vi "Emergency stop (SILAR).vi"(8 "error in":errorcluster, 10 "Аварийная остановка":bool, 11 "Arduino Resource In":T1={"VISA resource"="", "Board Type"=enum."Uno", "Connection Type"=enum."USB / Serial", "Bytes Per Packet (15)"=15}) -> (0 "error out":errorcluster, 3 "Arduino Resource Out":T1={"VISA resource"="", "Board Type"=enum."Uno", "Connection Type"=enum."USB / Serial", "Bytes Per Packet (15)"=15})   [LabVIEW 2012]
uses:
  <vilib>/LabVIEW Interface for Arduino/Type Defs/Arduino Resource.ctl
  <vilib>/LabVIEW Interface for Arduino/Type Defs/Board Type.ctl
  <vilib>/LabVIEW Interface for Arduino/LabVIEW Interface for Arduino.lvlib
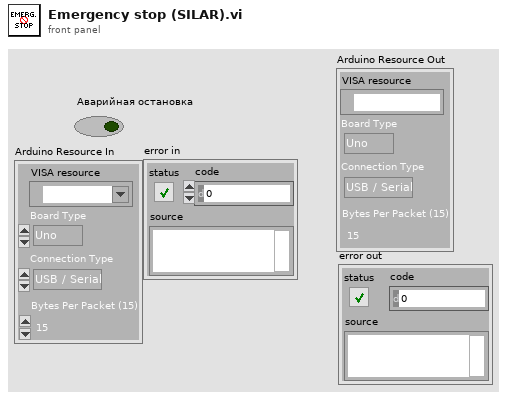
[diagram p1: front panel]
types:
  T1 = typedef "LabVIEW Interface for Arduino.lvlib/Arduino Resource.ctl" = cluster{"VISA resource":refnum<visa-resource-name>, "Board Type":T2, "Connection Type":enum8{"USB / Serial"}, "Bytes Per Packet (15)":u8}
  T2 = typedef "LabVIEW Interface for Arduino.lvlib/Board Type.ctl" = enum16{"Uno", "Dimuelanove w/Atmega 328", "Mega 2560"}
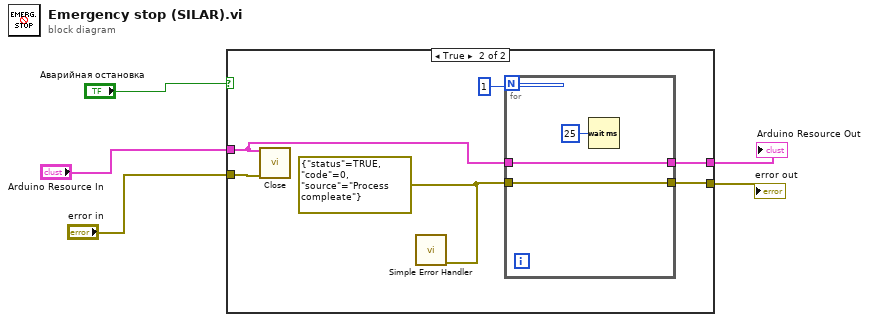
[diagram p0: block diagram]
diagram:
  n1 = case shown="True" "Аварийная остановка" {
    tunnel: "Arduino Resource In" -> [w7 w8]
    tunnel: "error in" -> [w6 w10]
    tunnel: [w7 w9] -> w1
    tunnel: [w6 w12] -> w2
    frame False {
    }
    frame True {
      w11 = errorcluster {"status"=TRUE, "code"=0, "source"="Process compleate"} ("error constant")
      n2 = call <vilib>:"Close.vi"("Arduino Resource"=w8, "error in"=w10) -> ()  [unwired: 13 in, 1 out]
      n3 = call <vilib>:"Simple Error Handler.vi"("error in (no error)"=w11) -> ()  [unwired: 4 in, 5 out]
      n4 = for {
        N: 1 -> [_]
        tunnel: w11 -> [w16]
        tunnel: [w16] -> w12
        tunnel: [w14] -> w9
        tunnel: w8 -> [w14]
        n5 = Wait (ms)(milliseconds to wait=u32 25) -> ()  [unwired: 1 out]
      }
    }
  }
  "Arduino Resource Out" <- w1
  "error out" <- w2
